vi "主板信息配置.vi"(3 "从板个数":dbl=3.0, 5 "主板信息查看":string[][](table)=[["电池额定容量", "0"], ["电池实际容量", "0"], ["SOC", "0"], ["SOH", "0"], ["产品编号", ""], ["车架(牌)号", ""], ["配置文件版本", ""], ["从板1电池节数", "10"], ["从板2电池节数", "10"], ["从板3电池节数", "10"], ["从板1温度个数", "2"], ["从板2温度个数", "2"], ["从板3温度个数", "2"]]) -> (0 "输出数组":string[][](array[string]), 1 "布尔":bool, 2 "从板个数 2":dbl)   [LabVIEW 2013]
panel:
  in  "个数":string
  in  "个数":string
  in  "自动计算通道电压":bool
  in  "通道电压清零":bool
  in  "清空":bool
  in  "电压全设":bool
  in  "温度全设":bool
  in  "计算起始值":bool
  in  "停止":bool
  in  "确定":bool
  in  "项目信息":T1
  in  "保险位置":bool[][](array[boolean])
  in  "主板信息":string[][](table)
  in  "20个通道电压个数":u8[](array[numeric]) max=12
  # "主板保险位置最多支持10个"
  # "1"
  # "2"
  # "3"
  # "4"
  # "5"
  # "6"
  # "7"
  # "8"
  # "9"
  # "10"
  # "11"
  # "12"
  # "第一通道"
  # "第二通道"
  # "第三通道"
  # "第四通道"
  # "第五通道"
  # "第六通道"
  # "第七通道"
  # "第八通道"
  # "第九通道"
  # "第十通道"
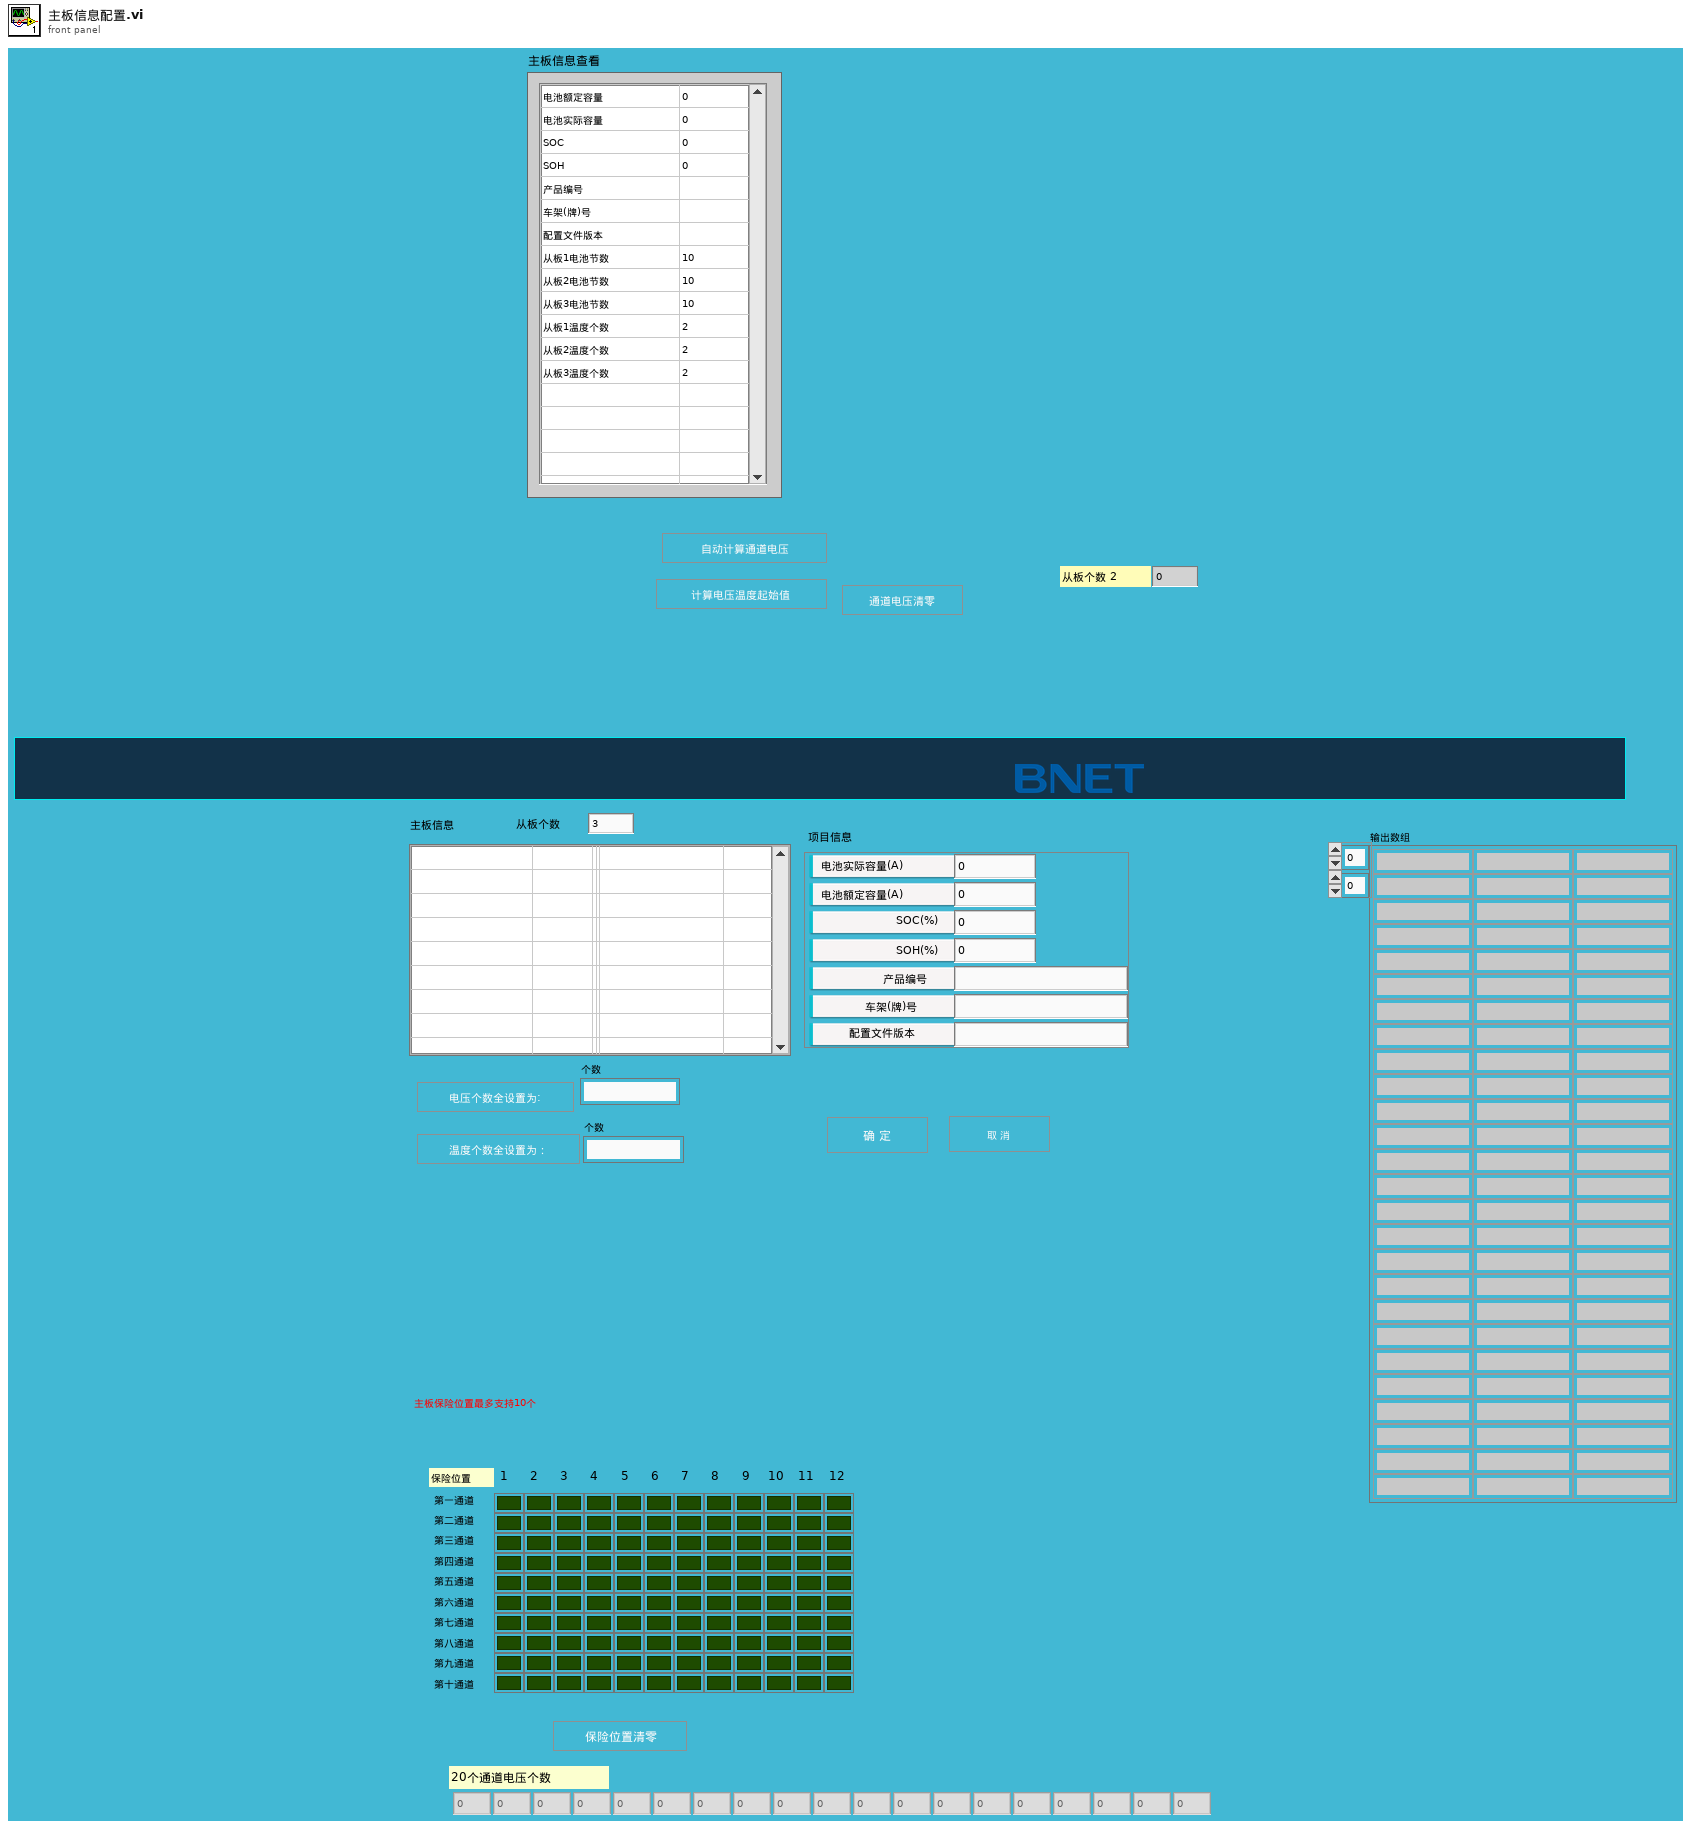
[diagram p1: front panel]
types:
  T1 = cluster{"电池额定容量(A)":dbl, "电池实际容量(A)":dbl, "SOC(%)":dbl, "SOH(%)":dbl, "产品编号":string, "车架(牌)号":string, "配置文件版本":string}
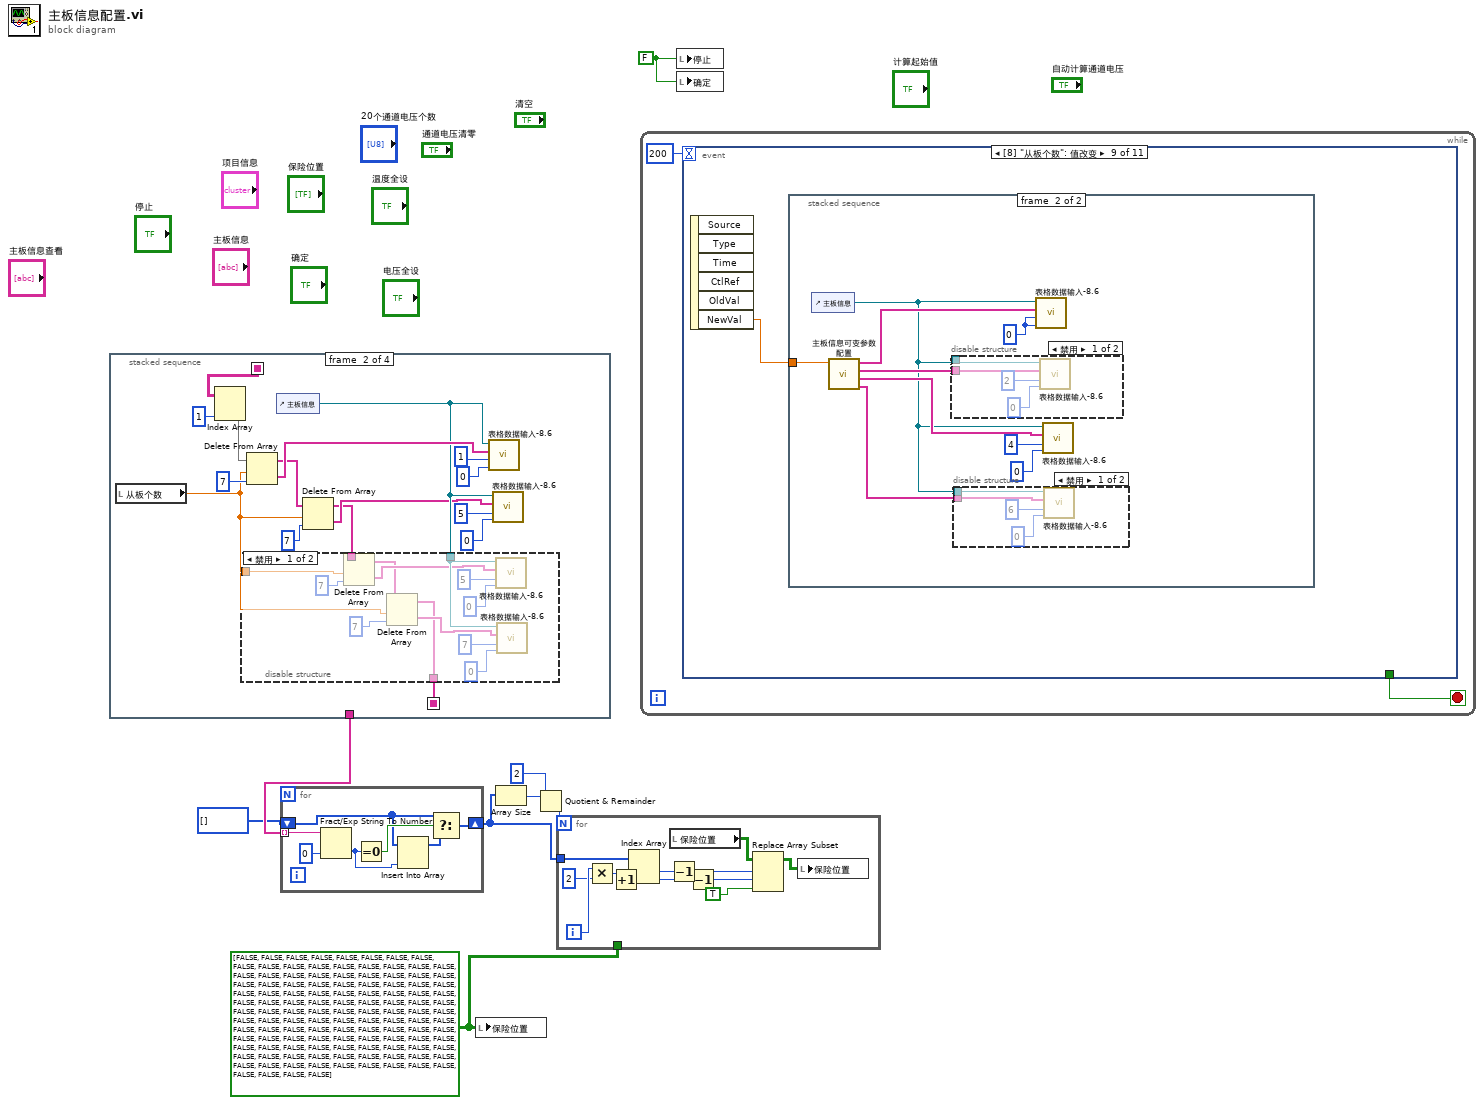
[diagram p0: block diagram]
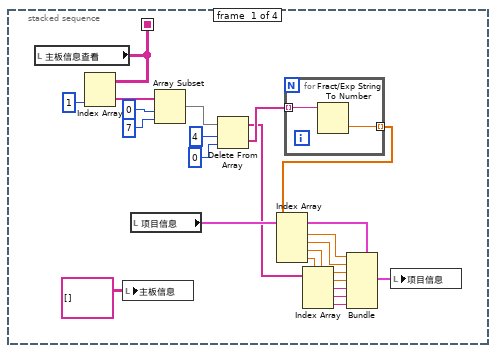
[diagram p2: hidden frame]
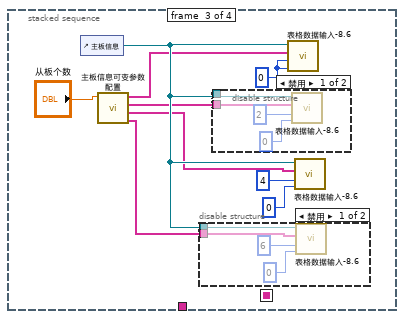
[diagram p4: hidden frame]
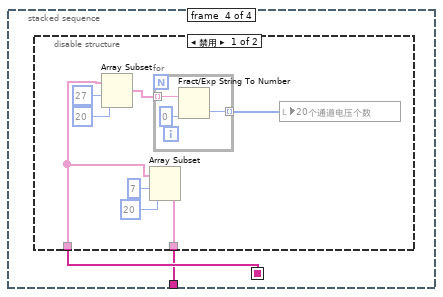
[diagram p7: hidden frame]
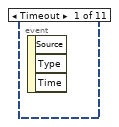
[diagram p9: hidden frame]
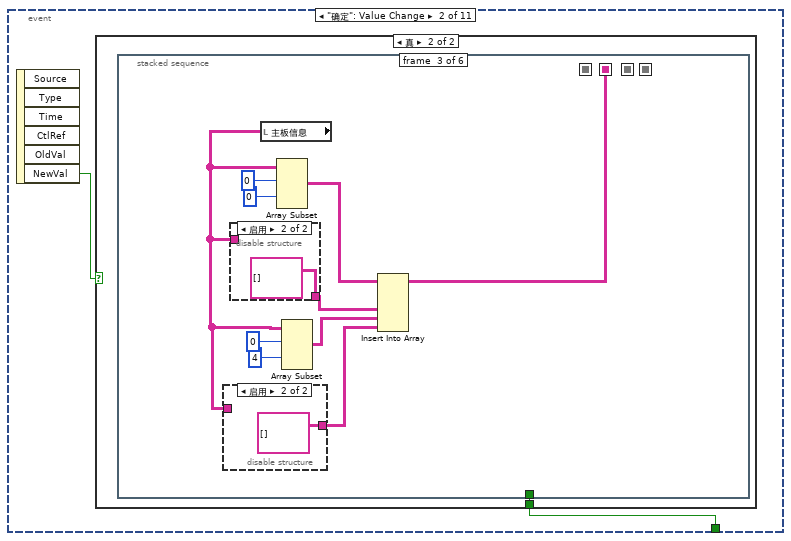
[diagram p10: hidden frame]
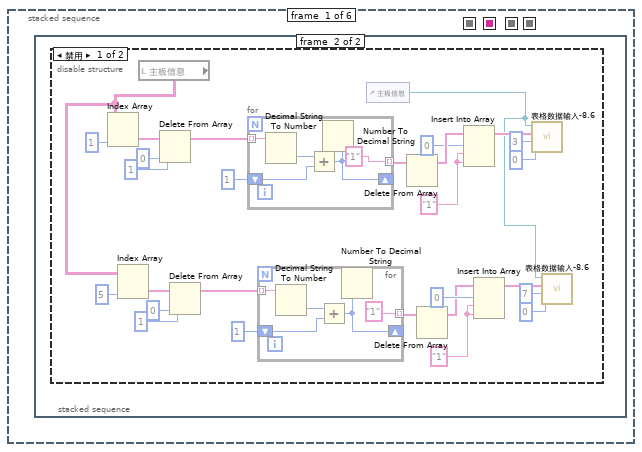
[diagram p12: hidden frame]
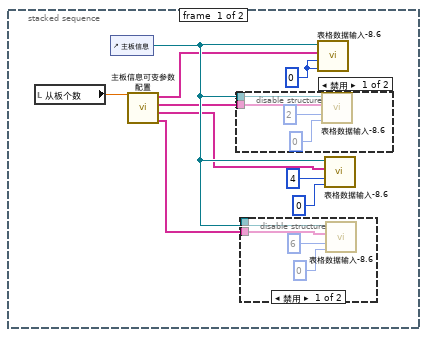
[diagram p13: hidden frame]
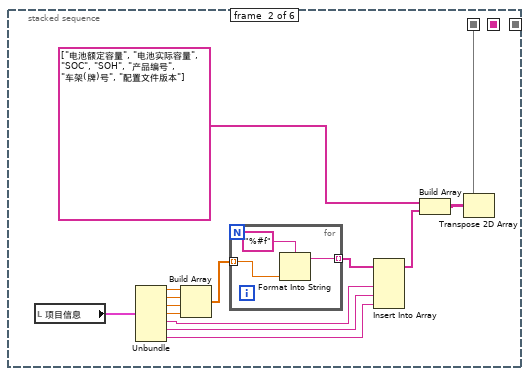
[diagram p17: hidden frame]
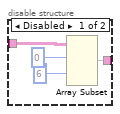
[diagram p18: hidden frame]
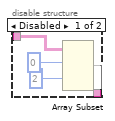
[diagram p19: hidden frame]
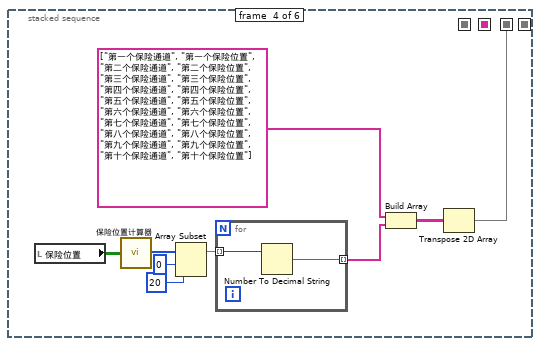
[diagram p20: hidden frame]
diagram:
  w2 = bool[][] [[FALSE, FALSE, FALSE, FALSE, FALSE, FALSE, FALSE, FALSE, FALSE, FALSE, FALSE, FALSE], [FALSE, FALSE, FALSE, FALSE, FALSE, FALSE, FALSE, FALSE, FALSE, FALSE, FALSE, FALSE], [FALSE, FALSE, FALSE, FALSE, FALSE, FALSE, FALSE, FALSE, FALSE, FALSE, FALSE, FALSE], [FALSE, FALSE, FALSE, FALSE, FALSE, FALSE, FALSE, FALSE, FALSE, FALSE, FALSE, FALSE], [FALSE, FALSE, FALSE, FALSE, FALSE, FALSE, FALSE, FALSE, FALSE, FALSE, FALSE, FALSE], [FALSE, FALSE, FALSE, FALSE, FALSE, FALSE, FALSE, FALSE, FALSE, FALSE, FALSE, FALSE], [FALSE, FALSE, FALSE, FALSE, FALSE, FALSE, FALSE, FALSE, FALSE, FALSE, FALSE, FALSE], [FALSE, FALSE, FALSE, FALSE, FALSE, FALSE, FALSE, FALSE, FALSE, FALSE, FALSE, FALSE], [FALSE, FALSE, FALSE, FALSE, FALSE, FALSE, FALSE, FALSE, FALSE, FALSE, FALSE, FALSE], [FALSE, FALSE, FALSE, FALSE, FALSE, FALSE, FALSE, FALSE, FALSE, FALSE, FALSE, FALSE]]
  w1 = FALSE ("取消按钮")
  n1 = stacked-sequence {
    seq-local: [w15 _ _ _] -> [_ w46 _ _]
    seq-local: [_ w33 _ _] -> [_ _ _ w79]
    tunnel: [_ _ _ w78] -> w8
    frame #0 {
      n2 = local read "主板信息查看"() -> (w15:string[][])
      n3 = Index Array(array=w15, index (col)=1 ("禁用的索引 (列)")) -> (element=w13:string[])  [unwired: 1 in]
      n4 = local write "主板信息"(string[][] [] ("主板信息")) -> ()
      n5 = local read "项目信息"() -> (w25:T1)
      n6 = Array Subset(array=w13, index=0 ("索引"), length=7 ("索引")) -> (w28:string[])
      n7 = Delete From Array(array=w28, length=4 ("长度"), index=0 ("索引 (行)")) -> (deleted portion=w26:string[], array with subset deleted=w10:string[])
      n8 = for {
        tunnel: w26 -> [w31] mode=indexing
        tunnel: [w30] -> w24 mode=indexing
        n9 = Fract/Exp String To Number(string=w31) -> (number=w30:dbl)  [unwired: 3 in, 1 out]
      }
      n10 = Index Array(array=w24) -> (element #1=w23:dbl, element #2=w22:dbl, element #3=w21:dbl, element #4=w20:dbl)  [unwired: 4 in]
      n11 = Index Array(array=w10) -> (element #1=w19:string, element #2=w18:string, element #3=w17:string)  [unwired: 3 in]
      n12 = Bundle(cluster=w25, "电池额定容量(A)"=w23, "电池实际容量(A)"=w22, "SOC(%)"=w21, "SOH(%)"=w20, "产品编号"=w19, "车架(牌)号"=w18, "配置文件版本"=w17) -> (w16:T1)
      n13 = local write "项目信息"(w16) -> ()
    }
    frame #1 {
      n14 = local read "从板个数"() -> (w32:dbl)
      n15 = Index Array(array=w46, index (col)=1 ("禁用的索引 (列)")) -> (element=w41:string[])  [unwired: 1 in]
      n16 = Delete From Array(array=w41, length=w32, index=7 ("索引")) -> (deleted portion=w39:string[], array with subset deleted=w37:string[])
      n17 = control-ref of="主板信息"() -> (w38:refnum<vi>)
      n18 = Delete From Array(array=w37, length=w32, index=7 ("索引")) -> (deleted portion=w35:string[], array with subset deleted=w34:string[])
      n19 = disable-structure shown="禁用" {
        disable-tunnel: w38 -> [w56 _]
        disable-tunnel: w34 -> [w55 _]
        disable-tunnel: [w49 _] -> w33
        disable-tunnel: w32 -> [w48 _]
        frame Disabled {
          n20 = Delete From Array(array=w55, length=w48, index=7 ("索引")) -> (deleted portion=w53:string[], array with subset deleted=w52:string[])
          n21 = Delete From Array(array=w52, length=w48, index=7 ("索引")) -> (deleted portion=w50:string[], array with subset deleted=w49:string[])
          n22 = call "表格数据输入-8.6.vi"("行数"=u32 0, "列数"=u32 5 ("行数"), "字符串数组"=w53, "表格引用"=w56) -> ()  [unwired: 8 in]
          n23 = call "表格数据输入-8.6.vi"("行数"=u32 0, "列数"=u32 7 ("行数"), "字符串数组"=w50, "表格引用"=w56) -> ()  [unwired: 8 in]
        }
        frame Enabled {
        }
      }
      n24 = call "表格数据输入-8.6.vi"("行数"=u32 0, "列数"=u32 1 ("行数"), "字符串数组"=w39, "表格引用"=w38) -> ()  [unwired: 8 in]
      n25 = call "表格数据输入-8.6.vi"("行数"=u32 0, "列数"=u32 5 ("行数"), "字符串数组"=w35, "表格引用"=w38) -> ()  [unwired: 8 in]
    }
    frame #2 {
      w63 = u32 0 ("行数")
      n26 = control-ref of="主板信息"() -> (w69:refnum<vi>)
      n27 = call "主板信息可变参数配置.vi"("从板个数"="从板个数") -> ("主板温度起始值"=w68:string[], "主板温度个数"=w67:string[], "主板电压起始值"=w64:string[], "电池节数"=w62:string[])  [unwired: 7 in]
      n28 = disable-structure shown="禁用" {
        disable-tunnel: w69 -> [w73 _]
        disable-tunnel: w68 -> [w72 _]
        frame Disabled {
          n29 = call "表格数据输入-8.6.vi"("行数"=u32 0, "列数"=u32 6 ("行数"), "字符串数组"=w72, "表格引用"=w73) -> ()  [unwired: 8 in]
        }
        frame Enabled {
        }
      }
      n30 = disable-structure shown="禁用" {
        disable-tunnel: w69 -> [w77 _]
        disable-tunnel: w64 -> [w75 _]
        frame Disabled {
          n31 = call "表格数据输入-8.6.vi"("行数"=u32 0, "列数"=u32 2 ("行数"), "字符串数组"=w75, "表格引用"=w77) -> ()  [unwired: 8 in]
        }
        frame Enabled {
        }
      }
      n32 = call "表格数据输入-8.6.vi"("行数"=w63, "列数"=w63, "字符串数组"=w62, "表格引用"=w69) -> ()  [unwired: 8 in]
      n33 = call "表格数据输入-8.6.vi"("行数"=u32 0, "列数"=u32 4 ("行数"), "字符串数组"=w67, "表格引用"=w69) -> ()  [unwired: 8 in]
    }
    frame #3 {
      n34 = disable-structure shown="禁用" {
        disable-tunnel: w79 -> [w81 _]
        disable-tunnel: [w80 _] -> w78
        frame Disabled {
          n35 = Array Subset(array=w81, index=27 ("索引"), length=20 ("索引")) -> (w86:string[])
          n36 = Array Subset(array=w81, index=7 ("索引"), length=20 ("索引")) -> (w80:string[])
          n37 = for {
            tunnel: w86 -> [w90] mode=indexing
            tunnel: [w89] -> w85 mode=indexing
            n38 = Fract/Exp String To Number(string=w90, default (0 dbl)=u8 0) -> (number=w89:u8)  [unwired: 2 in, 1 out]
          }
          n39 = local write "20个通道电压个数"(w85) -> ()
        }
        frame Enabled {
        }
      }
    }
  }
  n40 = for {
    tunnel: w8 -> [w97] mode=indexing
    shift-right: [w94] -> w4
    shift-left: i32[] [] -> [w93]
    n41 = Fract/Exp String To Number(string=w97, default (0 dbl)=u8 0) -> (number=w92:u8)  [unwired: 2 in, 1 out]
    n42 = Equal To 0?(x=w92) -> (x = 0?=w95:bool)
    n43 = Insert Into Array(array=w93, new element=w92) -> (w91:i32[])  [unwired: 1 in]
    n44 = Select(t=w93, s=w95, f=w91) -> (s? t:f=w94:i32[])
  }
  n45 = local write "保险位置"(w2) -> ()
  n46 = Array Size(array=w4) -> (size(s)=w6:i32)
  n47 = Quotient & Remainder(x=w6, y=2) -> (floor(x/y)=w3:i32)  [unwired: 1 out]
  n48 = for {
    N: w3 -> [_]
    tunnel: w4 -> [w109]
    tunnel: w2 -> [_]
    i -> [w108]
    n49 = Multiply(x=w108, y=2) -> (x*y=w106:i32)
    n50 = Increment(x=w106) -> (x+1=w105:i32)
    n51 = Index Array(array=w109, index #1=w106, index #2=w105) -> (element #1=w104:i32, element #2=w103:i32)
    n52 = Decrement(x=w104) -> (x-1=w101:i32)
    n53 = local read "保险位置"() -> (w99:bool[][])
    n54 = Decrement(x=w103) -> (x-1=w100:i32)
    n55 = Replace Array Subset(array=w99, new element=TRUE, index (row)=w101, index (col)=w100) -> (w98:bool[][])
    n56 = local write "保险位置"(w98) -> ()
  }
  n57 = while {
    stop <- w111 stop-if-true
    n58 = event shown="[8] \"从板个数\": 值改变" {
      selector: _ -> [_ _ _ _ _ _ _ _ _ _ _]
      dyn-events: _ -> [_ _ _ _ _ _ _ _ _ _ _]
      timeout: 200 -> [_ _ _ _ _ _ _ _ _ _ _]
      tunnel: [_ w112 _ _ _ _ _ _ _ w384 w389] -> w111
      event Timeout {
        n59 = event-data() -> ()  [unwired: 1 in, 3 out]
      }
      event "确定": Value Change {
        n60 = event-data() -> ("NewVal"=w113:bool)  [unwired: 1 in, 5 out]
        n61 = case shown="真" w113 {
          tunnel: [_ w114] -> w112
          frame False {
          }
          frame True {
            n62 = stacked-sequence {
              seq-local: [_ w170 _ _ _ _] -> [_ _ _ _ _ w232]
              seq-local: [_ _ w187 _ _ _] -> [_ _ _ _ _ w231]
              seq-local: [_ _ _ w210 _ _] -> [_ _ _ _ _ _]
              seq-local: [_ _ _ _ w221 _] -> [_ _ _ _ _ _]
              tunnel: [_ _ _ _ _ w229] -> w114
              frame #0 {
                n63 = stacked-sequence {
                  frame #0 {
                    w116 = u32 0 ("行数")
                    n64 = local read "从板个数"() -> (w123:dbl)
                    n65 = control-ref of="主板信息"() -> (w122:refnum<vi>)
                    n66 = call "主板信息可变参数配置.vi"("从板个数"=w123) -> ("主板温度起始值"=w121:string[], "主板温度个数"=w120:string[], "主板电压起始值"=w117:string[], "电池节数"=w115:string[])  [unwired: 7 in]
                    n67 = disable-structure shown="禁用" {
                      disable-tunnel: w122 -> [w131 _]
                      disable-tunnel: w117 -> [w129 _]
                      frame Disabled {
                        n68 = call "表格数据输入-8.6.vi"("行数"=u32 0, "列数"=u32 2 ("行数"), "字符串数组"=w129, "表格引用"=w131) -> ()  [unwired: 8 in]
                      }
                      frame Enabled {
                      }
                    }
                    n69 = disable-structure shown="禁用" {
                      disable-tunnel: w122 -> [w127 _]
                      disable-tunnel: w121 -> [w126 _]
                      frame Disabled {
                        n70 = call "表格数据输入-8.6.vi"("行数"=u32 0, "列数"=u32 6 ("行数"), "字符串数组"=w126, "表格引用"=w127) -> ()  [unwired: 8 in]
                      }
                      frame Enabled {
                      }
                    }
                    n71 = call "表格数据输入-8.6.vi"("行数"=w116, "列数"=w116, "字符串数组"=w115, "表格引用"=w122) -> ()  [unwired: 8 in]
                    n72 = call "表格数据输入-8.6.vi"("行数"=u32 0, "列数"=u32 4 ("行数"), "字符串数组"=w120, "表格引用"=w122) -> ()  [unwired: 8 in]
                  }
                  frame #1 {
                    n73 = disable-structure shown="禁用" {
                      frame Disabled {
                        w133 = "1"
                        w132 = "1"
                        n74 = local read "主板信息"() -> (w135:string[][])
                        n75 = Index Array(array=w135, index (col)=1 ("禁用的索引 (列)")) -> (element=w154:string[])  [unwired: 1 in]
                        n76 = Index Array(array=w135, index (col)=5 ("禁用的索引 (列)")) -> (element=w141:string[])  [unwired: 1 in]
                        n77 = Delete From Array(array=w154, length=1 ("长度"), index=0 ("索引")) -> (array with subset deleted=w153:string[])  [unwired: 1 out]
                        n78 = Delete From Array(array=w141, length=1 ("长度"), index=0 ("索引")) -> (array with subset deleted=w142:string[])  [unwired: 1 out]
                        n79 = for {
                          tunnel: w153 -> [w169] mode=indexing
                          shift-right: [w166] -> _
                          shift-left: 1 ("禁用的索引 (列)") -> [w167]
                          tunnel: ["1"] -> w158 mode=indexing
                          n80 = Decimal String To Number(string=w169) -> (number=w168:i32)  [unwired: 2 in, 1 out]
                          n81 = Add(x=w168, y=w167) -> (x+y=w166:i32)
                          n82 = Number To Decimal String(number=w166) -> ()  [unwired: 1 in, 1 out]
                        }
                        n83 = for {
                          tunnel: w142 -> [w164] mode=indexing
                          shift-right: [w161] -> _
                          shift-left: 1 ("禁用的索引 (列)") -> [w162]
                          tunnel: ["1"] -> w137 mode=indexing
                          n84 = Decimal String To Number(string=w164) -> (number=w163:i32)  [unwired: 2 in, 1 out]
                          n85 = Add(x=w163, y=w162) -> (x+y=w161:i32)
                          n86 = Number To Decimal String(number=w161) -> ()  [unwired: 1 in, 1 out]
                        }
                        n87 = control-ref of="主板信息"() -> (w134:refnum<vi>)
                        n88 = Delete From Array(array=w158) -> (array with subset deleted=w157:string[])  [unwired: 2 in, 1 out]
                        n89 = Delete From Array(array=w137) -> (array with subset deleted=w138:string[])  [unwired: 2 in, 1 out]
                        n90 = Insert Into Array(array=w157, index=0 ("索引"), new element #1=w132, new element #2=w132) -> (w150:string[])
                        n91 = Insert Into Array(array=w138, index=0 ("索引"), new element #1=w133, new element #2=w133) -> (w145:string[])
                        n92 = call "表格数据输入-8.6.vi"("行数"=u32 0, "列数"=u32 3, "字符串数组"=w150, "表格引用"=w134) -> ()  [unwired: 8 in]
                        n93 = call "表格数据输入-8.6.vi"("行数"=u32 0, "列数"=u32 7, "字符串数组"=w145, "表格引用"=w134) -> ()  [unwired: 8 in]
                      }
                      frame Enabled {
                      }
                    }
                  }
                }
              }
              frame #1 {
                n94 = local read "项目信息"() -> (w183:T1)
                n95 = Unbundle ("解除捆绑")(w183) -> ("电池额定容量(A)"=w181:dbl, "电池实际容量(A)"=w180:dbl, "SOC(%)"=w179:dbl, "SOH(%)"=w178:dbl, "产品编号"=w175:string, "车架(牌)号"=w174:string, "配置文件版本"=w173:string)
                n96 = Build Array(w181, w180, w179, w178) -> (w177:dbl[])
                n97 = for {
                  tunnel: w177 -> [w186] mode=indexing
                  tunnel: [w184] -> w176 mode=indexing
                  n98 = Format Into String(format string="%#f" ("格式字符串"), w186) -> (resulting string=w184:string)  [unwired: 2 in, 1 out]
                }
                n99 = Insert Into Array ("数组插入")(array=w176, new element #1=w175, new element #2=w174, new element #3=w173) -> (w172:string[])  [unwired: 1 in]
                n100 = Build Array ("创建数组")(string[] ["电池额定容量", "电池实际容量", "SOC", "SOH", "产品编号", "车架(牌)号", "配置文件版本"], w172) -> (w171:string[][])
                n101 = Transpose 2D Array ("二维数组转置")(2D array=w171) -> (transposed array=w170:string[][])
              }
              frame #2 {
                n102 = local read "主板信息"() -> (w192:string[][])
                n103 = disable-structure shown="启用" {
                  disable-tunnel: w192 -> [w198 _]
                  disable-tunnel: [w197 string[][] []] -> w188
                  frame Disabled {
                    n104 = Array Subset(array=w198, index (row)=0 ("索引"), index (col)=6 ("索引")) -> (w197:string[][])  [unwired: 2 in]
                  }
                  frame Enabled {
                  }
                }
                n105 = disable-structure shown="启用" {
                  disable-tunnel: w192 -> [w203 _]
                  disable-tunnel: [w202 string[][] []] -> w190
                  frame Disabled {
                    n106 = Array Subset(array=w203, index (row)=0 ("索引"), index (col)=2 ("索引")) -> (w202:string[][])  [unwired: 2 in]
                  }
                  frame Enabled {
                  }
                }
                n107 = Array Subset(array=w192, index (row)=0 ("索引"), index (col)=0 ("索引")) -> (w191:string[][])  [unwired: 2 in]
                n108 = Array Subset(array=w192, index (row)=0 ("索引"), index (col)=4 ("索引")) -> (w189:string[][])  [unwired: 2 in]
                n109 = Insert Into Array(array=w191, new element #1=w190, new element #2=w189, new element #3=w188) -> (w187:string[][])  [unwired: 2 in]
              }
              frame #3 {
                n110 = local read "保险位置"() -> (w215:bool[][])
                n111 = call "保险位置计算器.vi"("保险位置"=w215) -> ("输出数组"=w214:i32[])
                n112 = Array Subset(array=w214, index=0 ("索引"), length=20 ("长度")) -> (w209:i32[])
                n113 = for {
                  tunnel: w209 -> [w217] mode=indexing
                  tunnel: [w216] -> w213 mode=indexing
                  n114 = Number To Decimal String(number=w217) -> (decimal integer string=w216:string)  [unwired: 1 in]
                }
                n115 = Build Array(string[] ["第一个保险通道", "第一个保险位置", "第二个保险通道", "第二个保险位置", "第三个保险通道", "第三个保险位置", "第四个保险通道", "第四个保险位置", "第五个保险通道", "第五个保险位置", "第六个保险通道", "第六个保险位置", "第七个保险通道", "第七个保险位置", "第八个保险通道", "第八个保险位置", "第九个保险通道", "第九个保险位置", "第十个保险通道", "第十个保险位置"], w213) -> (w211:string[][])
                n116 = Transpose 2D Array(2D array=w211) -> (transposed array=w210:string[][])
              }
              frame #4 {
                n117 = local read "20个通道电压个数"() -> (w225:u8[])
                n118 = Array Subset(array=w225, index=0 ("索引"), length=20 ("长度")) -> (w220:u8[])
                n119 = for {
                  tunnel: w220 -> [w227] mode=indexing
                  tunnel: [w226] -> w224 mode=indexing
                  n120 = Number To Decimal String(number=w227) -> (decimal integer string=w226:string)  [unwired: 1 in]
                }
                n121 = Build Array(string[] ["第1通道电压个数", "第2通道电压个数", "第3通道电压个数", "第4通道电压个数", "第5通道电压个数", "第6通道电压个数", "第7通道电压个数", "第8通道电压个数", "第9通道电压个数", "第10通道电压个数", "第11通道电压个数", "第12通道电压个数", "第13通道电压个数", "第14通道电压个数", "第15通道电压个数", "第16通道电压个数", "第17通道电压个数", "第18通道电压个数", "第19通道电压个数", "第20通道电压个数"], w224) -> (w222:string[][])
                n122 = Transpose 2D Array(2D array=w222) -> (transposed array=w221:string[][])
              }
              frame #5 {
                n123 = local read "从板个数"() -> (→"从板个数 2":dbl)
                n124 = Insert Into Array(array=w232, new element=w231) -> (w230:string[][])  [unwired: 2 in]
                n125 = stacked-sequence {
                  tunnel: w230 -> [w234]
                  tunnel: [TRUE] -> w229
                  frame #0 {
                    "输出数组" <- w234
                  }
                }
                "布尔" <- w229
              }
            }
          }
        }
      }
      event "自动计算通道电压": Value Change {
        n126 = event-data() -> ("NewVal"=w235:bool)  [unwired: 1 in, 5 out]
        n127 = case shown="真" w235 {
          frame False {
          }
          frame True {
            n128 = local read "主板信息"() -> (w237:string[][])
            n129 = Index Array(array=w237, index (col)=1 ("禁用的索引 (列)")) -> (element=w239:string[])  [unwired: 1 in]
            n130 = Index Array(array=w239, index=0 ("索引")) -> (element=w241:string)
            n131 = Decimal String To Number(string=w241) -> (number=w242:i32)  [unwired: 2 in, 1 out]
            n132 = while {
              shift-right: [w251] -> _
              shift-left: w242 -> [w245]
              tunnel: [w249] -> w243 mode=indexing
              i -> [w258]
              stop <- w252 stop-if-true
              w247 = 12 ("y")
              n133 = local read "保险位置"() -> (w248:bool[][])
              n134 = Less?(x=w245, y=w247) -> (x < y?=w246:bool)
              n135 = Subtract(x=w245, y=w247) -> (x-y=w254:i32)
              n136 = Index Array(array=w248, index (row)=w258) -> (element=w257:bool[])  [unwired: 1 in]
              n137 = for {
                N: 12 -> [_]
                tunnel: w257 -> [w267] mode=indexing
                shift-right: [w268] -> w250
                shift-left: 0 -> [w265]
                n138 = Increment(x=w265) -> (x+1=w266:i32)
                n139 = Select(t=w266, s=w267, f=w265) -> (s? t:f=w268:i32)
              }
              n140 = Add(x=w254, y=w250) -> (x+y=w251:i32)
              n141 = case shown="假" w246 {
                tunnel: w250 -> [w261 w264]
                tunnel: [w260 w262] -> w249
                tunnel: w247 -> [w259 _]
                tunnel: w245 -> [_ w263]
                frame False {
                  n142 = Subtract(x=w259, y=w261) -> (x-y=w260:i32)
                }
                frame True {
                  n143 = Subtract(x=w263, y=w264) -> (x-y=w262:i32)
                }
              }
              n144 = Less Or Equal?(x=w251, y=0) -> (x <= y?=w252:bool)
            }
            n145 = Reshape Array(w243, 20 ("维数大小")) -> (w236:i32[])
            n146 = local write "20个通道电压个数"(w236) -> ()
          }
        }
      }
      event "清空": Value Change {
        n147 = event-data() -> ("NewVal"=w269:bool)  [unwired: 1 in, 5 out]
        n148 = case shown="真" w269 {
          frame False {
          }
          frame True {
            n149 = local write "保险位置"(bool[][] []) -> ()
          }
        }
      }
      event "通道电压清零": Value Change {
        n150 = event-data() -> ("NewVal"=w271:bool)  [unwired: 1 in, 5 out]
        n151 = case shown="真" w271 {
          frame False {
          }
          frame True {
            n152 = local write "20个通道电压个数"(i32[] [0, 0, 0, 0, 0, 0, 0, 0, 0, 0, 0, 0, 0, 0, 0, 0, 0, 0, 0, 0, 0] ("20个通道电压个数")) -> ()
          }
        }
      }
      event "计算起始值": Value Change {
        n153 = event-data() -> ("NewVal"=w273:bool)  [unwired: 1 in, 5 out]
        n154 = case shown="真" w273 {
          frame False {
          }
          frame True {
            n155 = stacked-sequence {
              frame #0 {
                w275 = u32 0 ("行数")
                n156 = local read "从板个数"() -> (w286:dbl)
                n157 = control-ref of="主板信息"() -> (w285:refnum<vi>)
                n158 = call "主板信息可变参数配置.vi"("从板个数"=w286) -> ("主板温度起始值"=w284:string[], "主板温度个数"=w281:string[], "主板电压起始值"=w277:string[], "电池节数"=w274:string[])  [unwired: 7 in]
                n159 = call "表格数据输入-8.6.vi"("行数"=w275, "列数"=w275, "字符串数组"=w274, "表格引用"=w285) -> ()  [unwired: 8 in]
                n160 = call "表格数据输入-8.6.vi"("行数"=u32 0, "列数"=u32 2 ("行数"), "字符串数组"=w277, "表格引用"=w285) -> ()  [unwired: 8 in]
                n161 = call "表格数据输入-8.6.vi"("行数"=u32 0, "列数"=u32 4 ("行数"), "字符串数组"=w281, "表格引用"=w285) -> ()  [unwired: 8 in]
                n162 = call "表格数据输入-8.6.vi"("行数"=u32 0, "列数"=u32 6 ("行数"), "字符串数组"=w284, "表格引用"=w285) -> ()  [unwired: 8 in]
              }
              frame #1 {
                w288 = "1"
                w287 = "1"
                n163 = local read "主板信息"() -> (w290:string[][])
                n164 = Index Array(array=w290, index (col)=1 ("禁用的索引 (列)")) -> (element=w309:string[])  [unwired: 1 in]
                n165 = Index Array(array=w290, index (col)=5 ("禁用的索引 (列)")) -> (element=w296:string[])  [unwired: 1 in]
                n166 = Delete From Array(array=w309, length=1 ("长度"), index=0 ("索引")) -> (array with subset deleted=w308:string[])  [unwired: 1 out]
                n167 = Delete From Array(array=w296, length=1 ("长度"), index=0 ("索引")) -> (array with subset deleted=w297:string[])  [unwired: 1 out]
                n168 = for {
                  tunnel: w308 -> [w324] mode=indexing
                  shift-right: [w321] -> _
                  shift-left: 1 ("禁用的索引 (列)") -> [w322]
                  tunnel: ["1"] -> w313 mode=indexing
                  n169 = Decimal String To Number(string=w324) -> (number=w323:i32)  [unwired: 2 in, 1 out]
                  n170 = Add(x=w323, y=w322) -> (x+y=w321:i32)
                  n171 = Number To Decimal String(number=w321) -> ()  [unwired: 1 in, 1 out]
                }
                n172 = for {
                  tunnel: w297 -> [w319] mode=indexing
                  shift-right: [w316] -> _
                  shift-left: 1 ("禁用的索引 (列)") -> [w317]
                  tunnel: ["1"] -> w292 mode=indexing
                  n173 = Decimal String To Number(string=w319) -> (number=w318:i32)  [unwired: 2 in, 1 out]
                  n174 = Add(x=w318, y=w317) -> (x+y=w316:i32)
                  n175 = Number To Decimal String(number=w316) -> ()  [unwired: 1 in, 1 out]
                }
                n176 = control-ref of="主板信息"() -> (w289:refnum<vi>)
                n177 = Delete From Array(array=w313) -> (array with subset deleted=w312:string[])  [unwired: 2 in, 1 out]
                n178 = Delete From Array(array=w292) -> (array with subset deleted=w293:string[])  [unwired: 2 in, 1 out]
                n179 = Insert Into Array(array=w312, index=0 ("索引"), new element #1=w287, new element #2=w287) -> (w305:string[])
                n180 = Insert Into Array(array=w293, index=0 ("索引"), new element #1=w288, new element #2=w288) -> (w300:string[])
                n181 = call "表格数据输入-8.6.vi"("行数"=u32 0, "列数"=u32 3, "字符串数组"=w305, "表格引用"=w289) -> ()  [unwired: 8 in]
                n182 = call "表格数据输入-8.6.vi"("行数"=u32 0, "列数"=u32 7, "字符串数组"=w300, "表格引用"=w289) -> ()  [unwired: 8 in]
              }
            }
          }
        }
      }
      event "温度全设": Value Change {
        n183 = event-data() -> ("NewVal"=w325:bool)  [unwired: 1 in, 5 out]
        n184 = case shown="真" w325 {
          frame False {
          }
          frame True {
            n185 = case shown="真" TRUE {
              tunnel: "个数" -> [_ w331]
              frame False {
              }
              frame True {
                n186 = local read "从板个数"() -> (w332:dbl)
                n187 = for {
                  N: w332 -> [_]
                  tunnel: w331 -> [w344]
                  tunnel: [w344] -> w329 mode=indexing
                  tunnel: [w343] -> w330 mode=indexing
                  n188 = Decimal String To Number(string=w344) -> (number=w343:i32)  [unwired: 2 in, 1 out]
                }
                n189 = control-ref of="主板信息"() -> (w333:refnum<vi>)
                n190 = disable-structure shown="启用" {
                  disable-tunnel: w330 -> [w341 _]
                  disable-tunnel: w329 -> [w339 w342]
                  disable-tunnel: [w336 w342] -> w328
                  frame Disabled {
                    n191 = Add Array Elements(numeric array=w341) -> (sum=w340:i32)
                    n192 = Number To Decimal String(number=w340) -> (decimal integer string=w338:string)  [unwired: 1 in]
                    n193 = Insert Into Array(array=w339, index=0 ("索引"), new element=w338) -> (w336:string[])
                  }
                  frame Enabled {
                  }
                }
                n194 = call "表格数据输入-8.6.vi"("行数"=u32 0, "列数"=u32 5, "字符串数组"=w328, "表格引用"=w333) -> ()  [unwired: 8 in]
              }
            }
          }
        }
      }
      event "电压全设": Value Change {
        n195 = event-data() -> ("NewVal"=w345:bool)  [unwired: 1 in, 5 out]
        n196 = case shown="真" w345 {
          frame False {
          }
          frame True {
            n197 = case shown="真" TRUE {
              tunnel: "个数" -> [_ w351]
              frame False {
              }
              frame True {
                n198 = local read "从板个数"() -> (w352:dbl)
                n199 = for {
                  N: w352 -> [_]
                  tunnel: w351 -> [w364]
                  tunnel: [w364] -> w349 mode=indexing
                  tunnel: [w363] -> w350 mode=indexing
                  n200 = Decimal String To Number(string=w364) -> (number=w363:i32)  [unwired: 2 in, 1 out]
                }
                n201 = control-ref of="主板信息"() -> (w353:refnum<vi>)
                n202 = disable-structure shown="启用" {
                  disable-tunnel: w350 -> [w361 _]
                  disable-tunnel: w349 -> [w359 w362]
                  disable-tunnel: [w356 w362] -> w348
                  frame Disabled {
                    n203 = Add Array Elements(numeric array=w361) -> (sum=w360:i32)
                    n204 = Number To Decimal String(number=w360) -> (decimal integer string=w358:string)  [unwired: 1 in]
                    n205 = Insert Into Array(array=w359, index=0 ("索引"), new element=w358) -> (w356:string[])
                  }
                  frame Enabled {
                  }
                }
                n206 = call "表格数据输入-8.6.vi"("行数"=u32 0, "列数"=u32 1, "字符串数组"=w348, "表格引用"=w353) -> ()  [unwired: 8 in]
              }
            }
          }
        }
      }
      event "从板个数": Value Change {
        n207 = event-data() -> ("NewVal"=w365:dbl)  [unwired: 1 in, 5 out]
        n208 = stacked-sequence {
          tunnel: w365 -> [_ w375]
          frame #0 {
            n209 = local write "主板信息"(string[][] [] ("主板信息可变参数（根据从板个数多少变化）")) -> ()
          }
          frame #1 {
            w373 = u32 0 ("行数")
            n210 = control-ref of="主板信息"() -> (w367:refnum<vi>)
            n211 = call "主板信息可变参数配置.vi"("从板个数"=w375) -> ("主板温度起始值"=w368:string[], "主板温度个数"=w369:string[], "主板电压起始值"=w372:string[], "电池节数"=w374:string[])  [unwired: 7 in]
            n212 = disable-structure shown="禁用" {
              disable-tunnel: w372 -> [w378 _]
              disable-tunnel: w367 -> [w376 _]
              frame Disabled {
                n213 = call "表格数据输入-8.6.vi"("行数"=u32 0, "列数"=u32 2 ("行数"), "字符串数组"=w378, "表格引用"=w376) -> ()  [unwired: 8 in]
              }
              frame Enabled {
              }
            }
            n214 = disable-structure shown="禁用" {
              disable-tunnel: w368 -> [w381 _]
              disable-tunnel: w367 -> [w380 _]
              frame Disabled {
                n215 = call "表格数据输入-8.6.vi"("行数"=u32 0, "列数"=u32 6 ("行数"), "字符串数组"=w381, "表格引用"=w380) -> ()  [unwired: 8 in]
              }
              frame Enabled {
              }
            }
            n216 = call "表格数据输入-8.6.vi"("行数"=w373, "列数"=w373, "字符串数组"=w374, "表格引用"=w367) -> ()  [unwired: 8 in]
            n217 = call "表格数据输入-8.6.vi"("行数"=u32 0, "列数"=u32 4 ("行数"), "字符串数组"=w369, "表格引用"=w367) -> ()  [unwired: 8 in]
          }
        }
      }
      event "停止": Value Change {
        n218 = event-data() -> ()  [unwired: 1 in, 6 out]
        n219 = stacked-sequence {
          tunnel: [TRUE] -> w384
          frame #0 {
            n220 = local write "输出数组"(string[][] [] ("输出数组")) -> ()
            n221 = local write "布尔"(FALSE ("布尔")) -> ()
          }
        }
      }
      event Panel Close? {
        n222 = event-data() -> ()  [unwired: 1 in, 4 out]
        n223 = stacked-sequence {
          tunnel: [TRUE] -> w389
          frame #0 {
            n224 = local write "输出数组"(string[][] [] ("输出数组")) -> ()
            n225 = local write "布尔"(FALSE ("布尔")) -> ()
          }
        }
        n226 = event-data("Discard?"=FALSE ("放弃？")) -> ()  [unwired: 1 in, 1 out]
      }
    }
  }
  n227 = local write "停止"(w1) -> ()
  n228 = local write "确定"(w1) -> ()
